vi "kvCanWriteMsgFlag.vi"(4 "Error Frame":bool, 5 "Wakeup":bool, 6 "Single Shot":bool, 7 "Remote Request":bool, 8 "Bit Rate Switch":bool, 9 "FD Frame":bool, 10 "Extended 29-bit Id":bool, 11 "Standard 11-bit Id":bool) -> (3 "Flag Value":u32)   [LabVIEW 2022 SP3]
doc: "This VI translates the write message flags into the numeric value used by the KVaser CANLib.\n\nThis should never be used in an application, but is an internal VI."
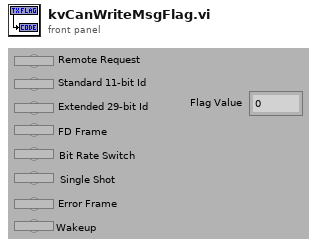
[diagram p1: front panel]
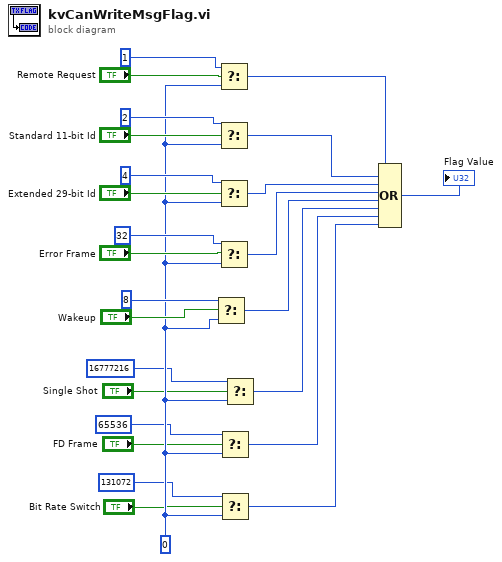
[diagram p0: block diagram]
diagram:
  w10 = u32 0
  n1 = Select(t=u32 8, s="Wakeup", f=w10) -> (s? t:f=w11:u32)
  n2 = Select(t=u32 1, s="Remote Request", f=w10) -> (s? t:f=w18:u32)
  n3 = Select(t=u32 2, s="Standard 11-bit Id", f=w10) -> (s? t:f=w17:u32)
  n4 = Select(t=u32 4, s="Extended 29-bit Id", f=w10) -> (s? t:f=w16:u32)
  n5 = Select(t=u32 32, s="Error Frame", f=w10) -> (s? t:f=w15:u32)
  n6 = Select(t=u32 65536, s="FD Frame", f=w10) -> (s? t:f=w8:u32)
  n7 = Select(t=u32 131072, s="Bit Rate Switch", f=w10) -> (s? t:f=w7:u32)
  n8 = Select(t=u32 16777216, s="Single Shot", f=w10) -> (s? t:f=w9:u32)
  n9 = Compound Arithmetic op=OR(w18, w17, w16, w15, w11, w9, w8, w7) -> (→"Flag Value":u32)
